vi "Agilent N6700 Series Configure Staircase Waveform.vi"() -> ()   [LabVIEW 2016]
doc: "Configures a staircase waveform.\n\n<b>Note:</b>\n\nThis VI only applies to the N6705B and N6705C DC Power Analyzer."
uses:
  <instrlib>/Agilent N6700 Series/Public/Configuration/Waveform/Configure Waveform (Staircase).vi
  <instrlib>/Agilent N6700 Series/Agilent N6700 Series.lvlib
panel:
  in  "Waveform Last Termination (False: Off)":bool
  in  "Waveform Count (10)":i32=1
  in  "Staircase End Level (5.0)":dbl=5.0 format="%^.3e"
  in  "Staircase End Time (2.0 s)":dbl=2.0 format="%^.3e"
  in  "Staircase Total Time (1.0 s)":dbl=3.0 format="%^.3e"
  in  "Staircase Start Time (0.0 s)":dbl=2.0 format="%^.3e"
  in  "Staircase Start Level (0.0)":dbl format="%^.3e"
  in  "Staircase Steps (12)":i32=12
  in  "Channel Name (1)":string="1"
  in  "VISA resource name":refnum<visa-resource-name>
  # "(c) 2012-2019  National Instruments.  ALL RIGHTS RESERVED."
  # "Agilent N6705 DC Power Supply"
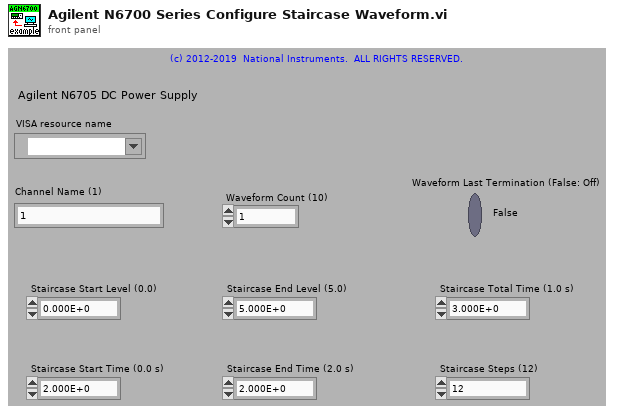
[diagram p1: front panel]
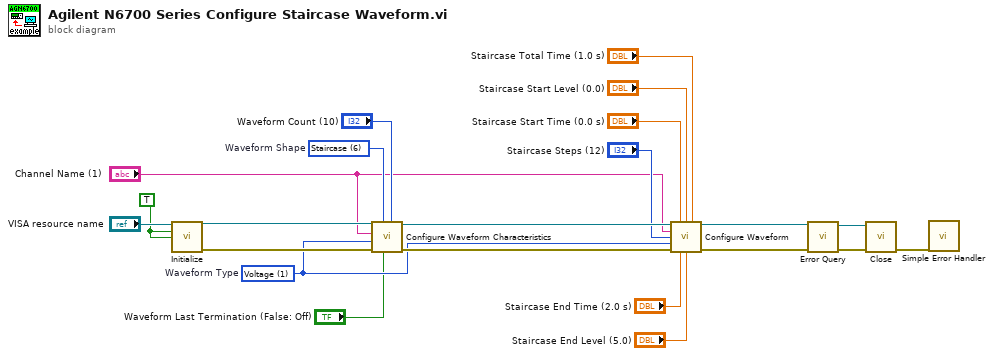
[diagram p0: block diagram]
diagram:
  w6 = 6 items=["None", "Constant Dwell", "Exponential", "Pulse", "Ramp", "Sine Wave", "Staircase", "Step", "Trapezoid", "Sequence", "User Defined"]  # Waveform Shape
  w12 = 1 items=["Voltage"=1, "Current"=0]  # Waveform Type
  w14 = TRUE ("Reset? (T: Yes)")
  n1 = call <instrlib>:"Initialize.vi"("VISA resource name"="VISA resource name", "ID Query? (T: Yes)"=w14, "Reset? (T: Yes)"=w14) -> ("VISA resource name out"=w16:refnum<visa-resource-name>, "error out"=w21:errorcluster)  [unwired: 11 in]
  n2 = call <instrlib>:"Configure Waveform Characteristics.vi"("Waveform Count (1)"="Waveform Count (10)", "Waveform Last Termination (False: Off)"="Waveform Last Termination (False: Off)", "Waveform Shape (0: None)"=w6, "error in (no error)"=w21, "Waveform Type (1: Voltage)"=w12, "Channel Name (1)"="Channel Name (1)", "VISA resource name"=w16) -> ("error out"=w20:errorcluster, "VISA resource name out"=w17:refnum<visa-resource-name>)  [unwired: 3 in]
  n3 = call-poly <instrlib>:"Configure Waveform.vi"("VISA resource name"=w17, "Staircase Start Time (0.0 s)"="Staircase Start Time (0.0 s)", "Staircase Start Level (0.0)"="Staircase Start Level (0.0)", "Staircase Total Time (1.0 s)"="Staircase Total Time (1.0 s)", "Channel Name (1)"="Channel Name (1)", "Staircase Steps (10)"="Staircase Steps (12)", "Waveform Type (1: Voltage)"=w12, "error in (no error)"=w20, "Staircase End Time (0.0 s)"="Staircase End Time (2.0 s)", "Staircase End Level (0.0)"="Staircase End Level (5.0)") -> ("VISA resource name out"=w4:refnum<visa-resource-name>, "error out"=w3:errorcluster)  [unwired: 4 in]
  n4 = call <instrlib>:"Error Query.vi"("VISA resource name"=w4, "error in (no error)"=w3) -> ("VISA resource name out"=w18:refnum<visa-resource-name>, "error out"=w19:errorcluster)  [unwired: 10 in, 2 out]
  n5 = call <instrlib>:"Close.vi"("VISA resource name"=w18, "error in (no error)"=w19) -> ("error out"=w22:errorcluster)  [unwired: 13 in]
  n6 = call <vilib>:"Simple Error Handler.vi"("error in (no error)"=w22) -> ()  [unwired: 4 in, 5 out]
